vi "Read Mixed Module.vi"(0 "IOV ref in":T7, 1 "R/W Case":T2, 3 "Channel Type":T6, 5 "Output Data in":T3 {"BD Refs"."Data Reference" format="%.0x"}, 9 "Output FIFO buffer in":dbl[](array[numeric]), 11 "error in (no error)":errorcluster, 12 "Mixed IO in":T1) -> (4 "IOV ref out":T7, 6 "Output Data out":T3 {"BD Refs"."Data Reference" format="%.0x"}, 10 "Output FIFO buffer out":dbl[](array[numeric]), 14 "Mixed IO out":T1, 15 "error out":errorcluster)   [LabVIEW 2011, in "Scan Engine Custom Device.lvlib"]
uses:
  Scan Engine Custom Device.lvlib
  Type Defs/Open Module IOVs.ctl
  Type Defs/Output Data.ctl
  <vilib>/NI Veristand/Custom Device API/Block Data Reference.ctl
  <vilib>/NI Veristand/Custom Device API/Data Reference.ctl
  Modules.lvlibp/RSI Module/Channel Type.ctl
  Type Defs/RW Case.ctl
  Type Defs/Mixed IO.ctl
  <vilib>/NI Veristand/Custom Device API/Global Data Refs.vi
  <vilib>/NI Veristand/Custom Device API/Custom Device API.lvlib
  Modules.lvlibp/RSI Module/RSI Module.lvclass
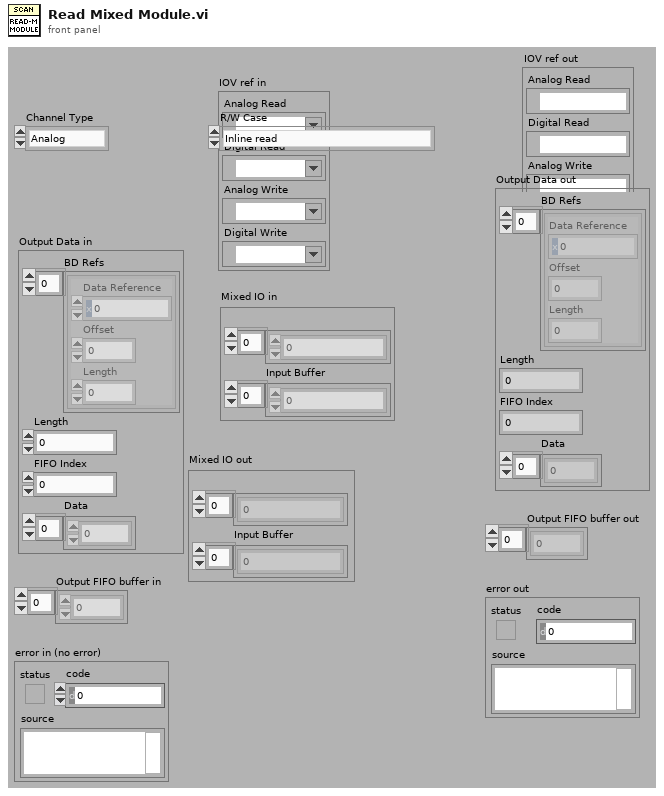
[diagram p1: front panel]
types:
  T1 = typedef "Scan Engine Custom Device.lvlib/Mixed IO.ctl" = cluster{"Input Channel Indices":i32[], "Input Buffer":dbl[]}
  T2 = typedef "Scan Engine Custom Device.lvlib/RW Case.ctl" = enum16{"Inline read", "Inline write", "Async - Inline loop read", "Async - Inline loop write", "Async loop (read/write)"}
  T3 = typedef "Scan Engine Custom Device.lvlib/Output Data.ctl" = cluster{"BD Refs":T4[], "Length":i32, "FIFO Index":i32, "Data":dbl[]}
  T4 = typedef "Custom Device API.lvlib/Block Data Reference.ctl" = cluster{"Data Reference":T5, "Offset":i32, "Length":i32}
  T5 = typedef "Custom Device API.lvlib/Data Reference.ctl" = i32
  T6 = typedef "Modules.lvlibp/RSI Module.lvclass/Channel Type.ctl" = enum16{"Analog", "Digital"}
  T7 = typedef "Scan Engine Custom Device.lvlib/Open Module IOVs.ctl" = cluster{"Analog Read":refnum<k21>, "Digital Read":refnum<k21>, "Analog Write":refnum<k21>, "Digital Write":refnum<k21>}
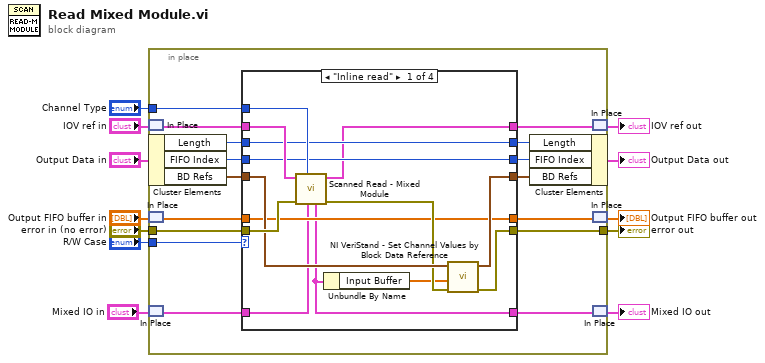
[diagram p0: block diagram]
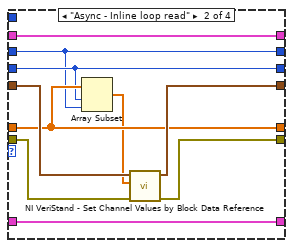
[diagram p2: hidden frame]
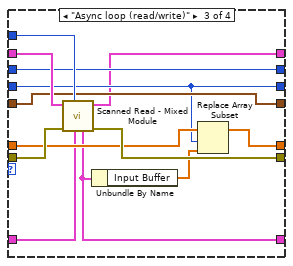
[diagram p3: hidden frame]
diagram:
  n1 = in-place {
    in-place-border: "R/W Case" -> [w28]
    in-place-border: "Channel Type" -> [w27]
    in-place-border: "error in (no error)" -> [w26]
    in-place-border: [w24] -> w1
    n2 = in-place-match #1("IOV ref in") -> (w14:T7)
    n3 = in-place-cluster #2("Output Data in") -> ("Length"=w19:i32, "FIFO Index"=w22:i32, "BD Refs"=w25:T4[])
    n4 = in-place-match #3("Output FIFO buffer in") -> (w18:dbl[])
    n5 = in-place-match #4("Mixed IO in") -> (w16:T1)
    n6 = case shown="\"Inline read\"" w28 {
      tunnel: w27 -> [w42 _ w65 _]
      tunnel: w14 -> [w41 w45 w64 w72]
      tunnel: w26 -> [w40 w51 w63 w67]
      tunnel: w18 -> [w35 w48 w60 w68]
      tunnel: w25 -> [w39 w52 w61 w69]
      tunnel: [w37 w50 w62 w67] -> w24
      tunnel: [w36 w49 w61 w69] -> w23
      tunnel: [w35 w48 w59 w68] -> w17
      tunnel: w22 -> [w34 w47 w58 w70]
      tunnel: [w34 w47 w58 w70] -> w21
      tunnel: [w33 w46 w57 w71] -> w20
      tunnel: [w32 w45 w56 w72] -> w13
      tunnel: w19 -> [w33 w46 w57 w71]
      tunnel: w16 -> [w31 w44 w55 w66]
      tunnel: [w30 w44 w54 w66] -> w15
      frame "Inline read" {
        n7 = call "Scanned Read - Mixed Module.vi"("Mixed IO in"=w31, "Channel Type"=w42, "error in (no error)"=w40, "IOV ref in"=w41) -> ("error out"=w38:errorcluster, "IOV ref out"=w32:T7, "Mixed IO out"=w30:T1)  [unwired: 5 in]
        n8 = Unbundle By Name(w30) -> ("Input Buffer"=w29:dbl[])
        n9 = call <vilib>:"NI VeriStand - Set Channel Values by Block Data Reference.vi"("error in (no error)"=w38, "Values Array in"=w29, "Block Data Ref"=w39) -> ("error out"=w37:errorcluster, "Block Data Ref dup"=w36:T4[])  [unwired: 6 in, 1 out]
      }
      frame "Async - Inline loop read" {
        n10 = Array Subset(array=w48, index=w47, length=w46) -> (w43:dbl[])
        n11 = call <vilib>:"NI VeriStand - Set Channel Values by Block Data Reference.vi"("error in (no error)"=w51, "Values Array in"=w43, "Block Data Ref"=w52) -> ("error out"=w50:errorcluster, "Block Data Ref dup"=w49:T4[])  [unwired: 6 in, 1 out]
      }
      frame "Async loop (read/write)" {
        n12 = call "Scanned Read - Mixed Module.vi"("Mixed IO in"=w55, "Channel Type"=w65, "error in (no error)"=w63, "IOV ref in"=w64) -> ("error out"=w62:errorcluster, "IOV ref out"=w56:T7, "Mixed IO out"=w54:T1)  [unwired: 5 in]
        n13 = Unbundle By Name(w54) -> ("Input Buffer"=w53:dbl[])
        n14 = Replace Array Subset(array=w60, new element=w53, index=w58) -> (w59:dbl[])
      }
      frame Default {
      }
    }
    n15 = in-place-cluster #2("Length"=w20, "FIFO Index"=w21, "BD Refs"=w23) -> (→"Output Data out":T3)
    n16 = in-place-match #1(w13) -> (→"IOV ref out":T7)
    n17 = in-place-match #3(w17) -> (→"Output FIFO buffer out":dbl[])
    n18 = in-place-match #4(w15) -> (→"Mixed IO out":T1)
  }
  "error out" <- w1
